vi "Set Data Name__ogtk.vi"(8 "error in (no error)":errorcluster, 9 "Data Name":string, 10 "Data":variant) -> (0 "error out":errorcluster, 2 "Renamed Data":variant)   [LabVIEW 2009]
doc: "Changes the Data Name of Variant Data.\n<b>Note:</b> Variant attributes will persist after this operation."
panel:
  # "Please visit http://www.OpenG.org to learn about the\nOpen Source LabVIEW software movement.\n\nNOTICE -- YOU MUST LEAVE THIS NOTICE IN PLACE.  PER THE TERMS OF THE LICENSE BELOW, YOU MAY SUBLICENSE THIS SOFTWARE \nIN ANY WAY THAT DOES NOT CONFLICT WITH THIS LICENSE.\n\n### BSD License (http://www.opensource.org/licenses/bsd-license.php) Begin ###\n \nCopyright (c) 2002, Jean-Pierre Drolet <drolet_jp@hotmail.com>\nCopyright (c) 2002-2006, Jim Kring <jim@jimkring.com>\nCopyright (c) 2011, Jonathon Green <jg@jgcode.net>\n\nAll rights reserved.\n\nRedistribution and use in source and binary forms, with or without modification, are permitted provided that the following conditions are met:\n\n    * Redistributions of source code must retain the above copyright notice, this list of conditions and the following disclaimer.\n    * Redistributions in binary form must reproduce the above copyright notice, this list of conditions and the following disclaimer in the \n       documentation and/or other materials provided with the distribution.\n    * Neither the name of SciWare, James Kring, Inc., nor the names of its contributors may be used to endorse or promote products derived \n       from this software without specific prior written permission.\n\nTHIS SOFTWARE IS PROVIDED BY THE COPYRIGHT HOLDERS AND CONTRIBUTORS \"AS IS\" AND ANY EXPRESS OR IMPLIED WARRANTIES, \nINCLUDING, BUT NOT LIMITED TO, THE IMPLIED WARRANTIES OF MERCHANTABILITY AND FITNESS FOR A PARTICULAR PURPOSE ARE \nDISCLAIMED. IN NO EVENT SHALL THE COPYRIGHT OWNER OR CONTRIBUTORS BE LIABLE FOR ANY DIRECT, INDIRECT, INCIDENTAL,\n SPECIAL, EXEMPLARY, OR CONSEQUENTIAL DAMAGES (INCLUDING, BUT NOT LIMITED TO, PROCUREMENT OF SUBSTITUTE GOODS OR \nSERVICES; LOSS OF USE, DATA, OR PROFITS; OR BUSINESS INTERRUPTION) HOWEVER CAUSED AND ON ANY THEORY OF LIABILITY, \nWHETHER IN CONTRACT, STRICT LIABILITY, OR TORT (INCLUDING NEGLIGENCE OR OTHERWISE) ARISING IN ANY WAY OUT OF THE USE \nOF THIS SOFTWARE, EVEN IF ADVISED OF THE POSSIBILITY OF SUCH DAMAGE.\n\n### BSD License End ###"
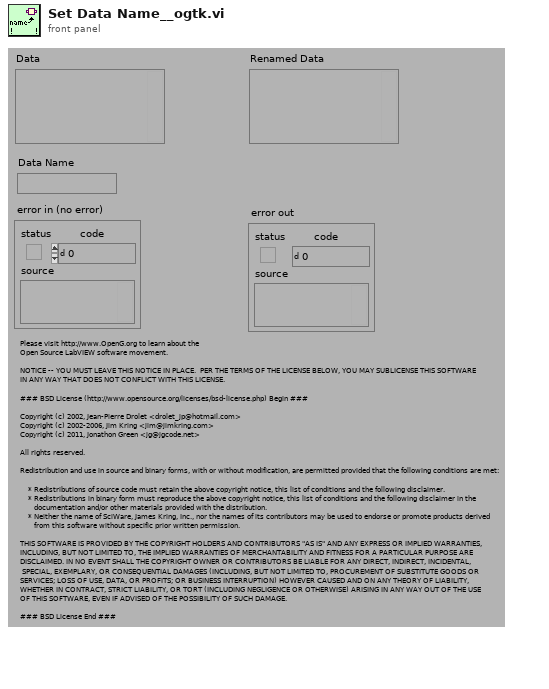
[diagram p1: front panel]
types:
  T1 = typedef "Type Descriptor Header__ogtk.ctl" = cluster{"length":u16, "private":u8, "type":T2, "# elements":u16}
  T2 = typedef "Type Descriptor Enumeration__ogtk.ctl" = enum8{"<Null>", "I8", "I16", "I32", "I64", "U8", "U16", "U32", "U64", "SGL", "DBL", "EXT", "CSG", "CDB", "CXT", "0x0F", "0x10", "0x11", "0x12", "0x13", "0x14", "Enum U8", "Enum U16", "Enum U32", "Enum U64", "SGL PQ", "DBL PQ", "EXT PQ", "CSG PQ", "CDB PQ", "CXT PQ", "0x1F", "0x20", "Boolean", "0x22", "0x23", "0x24", "0x25", "0x26", "0x27", "0x28", "0x29", "0x2A", "0x2B", "0x2C", "0x2D", "0x2E", "0x2F", "String", "0x31", "Path", "Pict", "0x34", "0x35", "0x36", "DAQ", "0x38", "0x39", "0x3A", "0x3B", "0x3C", "0x3D", "0x3E", "0x3F", "Array", "0x41", "0x42", "0x43", "0x44", "0x45", "0x46", "0x47", "0x48", "0x49", "0x4A", "0x4B", "0x4C", "0x4D", "0x4E", "0x4F", "Cluster", "0x51", "0x52", "Variant", "Waveform", "0x55", "0x56", "0x57", "0x58", "0x59", "0x5A", "0x5B", "0x5C", "0x5D", "0x5E", "0x5F", "0x60", "0x61", "0x62", "0x63", "0x64", "0x65", "0x66", "0x67", "0x68", "0x69", "0x6A", "0x6B", "0x6C", "0x6D", "0x6E", "0x6F", "Refnum"}
  T3 = typedef "Type Descriptor__ogtk.ctl" = i16[]
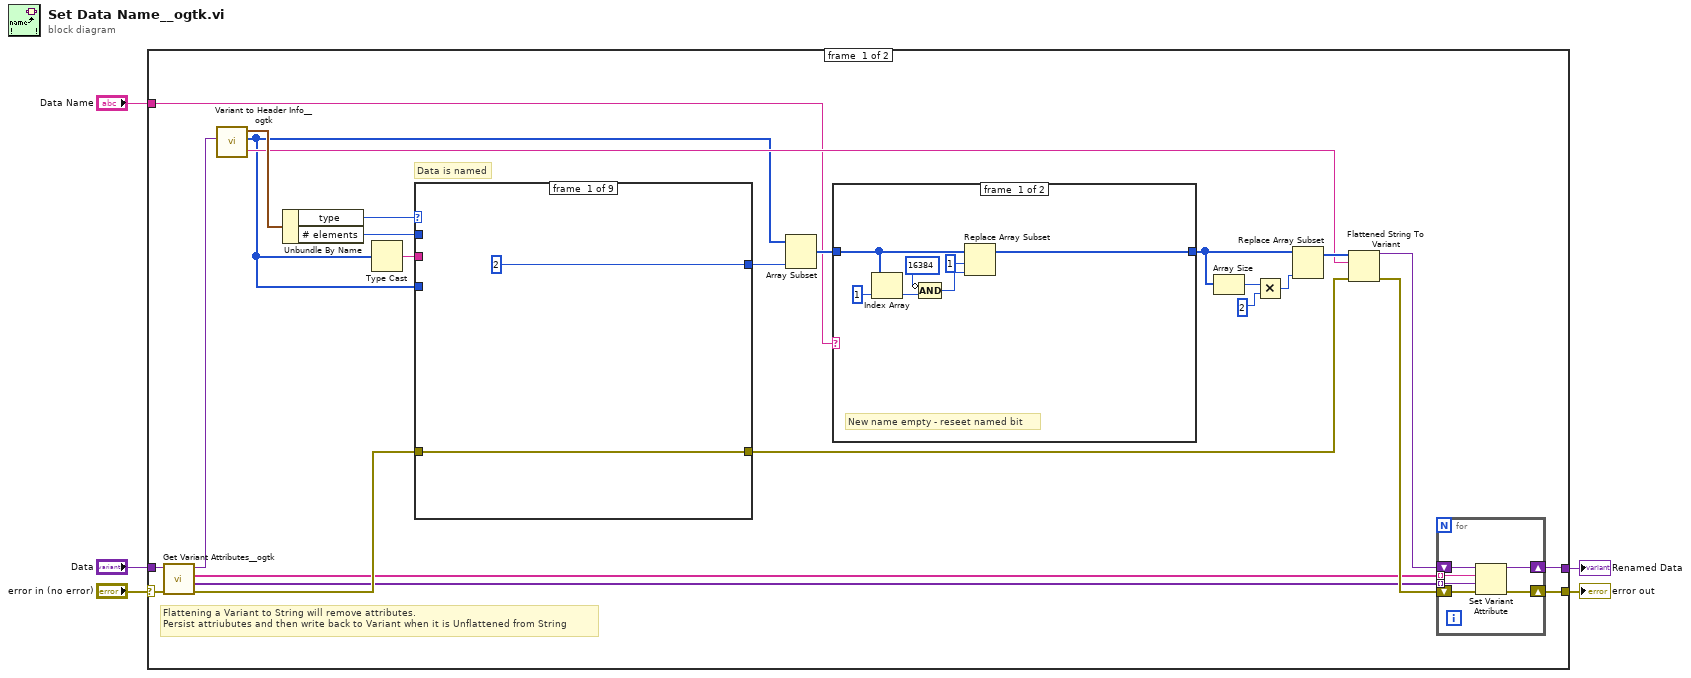
[diagram p0: block diagram]
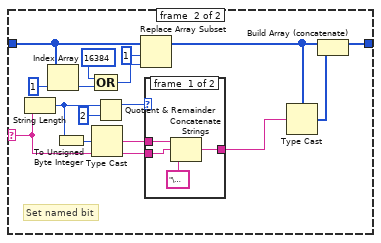
[diagram p2: hidden frame]
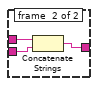
[diagram p3: hidden frame]
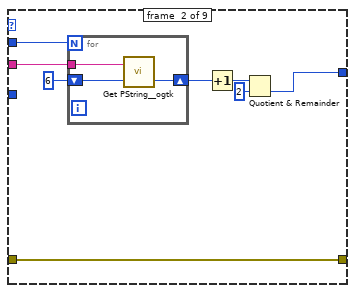
[diagram p4: hidden frame]
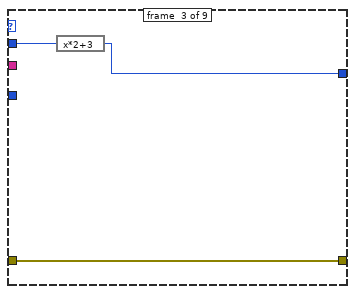
[diagram p5: hidden frame]
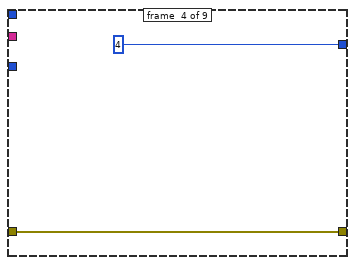
[diagram p6: hidden frame]
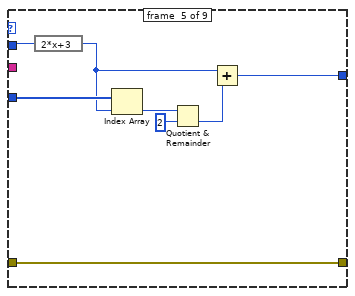
[diagram p7: hidden frame]
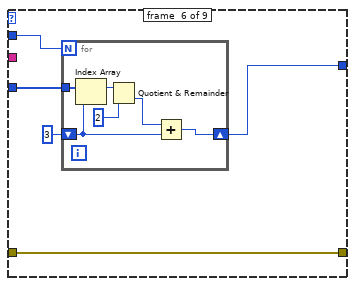
[diagram p8: hidden frame]
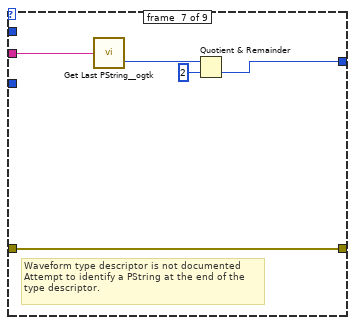
[diagram p9: hidden frame]
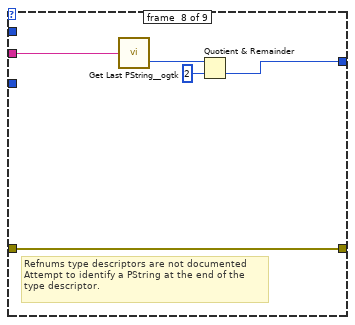
[diagram p10: hidden frame]
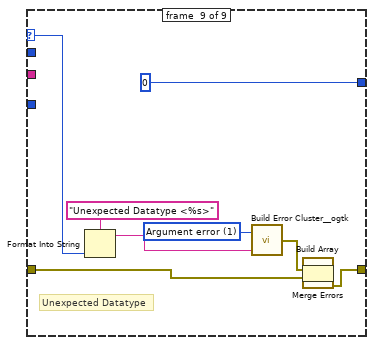
[diagram p11: hidden frame]
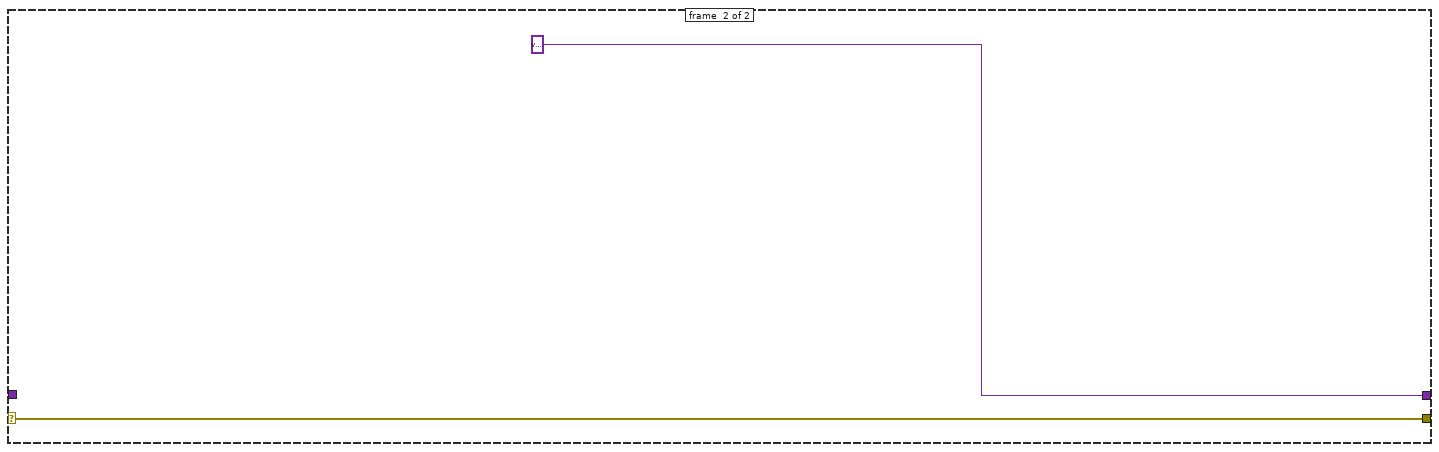
[diagram p12: hidden frame]
diagram:
  n1 = case shown="No Error" "error in (no error)" {
    selector: "error in (no error)" -> [w13 w124]
    tunnel: [w10 w124] -> w5
    tunnel: [w6 variant ("Renamed Data")] -> w3
    tunnel: "Data Name" -> [w16 _]
    tunnel: "Data" -> [w15 _]
    frame #0 {
      # "Flattening a Variant to String will remove attributes.\nPersist attriubutes and then write back to Variant when it is Unflattened from String"
      # "Data is named"
      n2 = call "Get Variant Attributes__ogtk.vi"("error in"=w13, "Variant"=w15) -> ("error out"=w12:errorcluster, "value(s)"=w9:variant[], "names"=w8:string[], "duplicate Variant"=w14:variant)  [unwired: 2 in]
      n3 = call "Variant to Header Info__ogtk.vi"("Variant"=w14) -> ("Type Descriptor Header"=w30:T1, "Type Descriptor"=w17:T3, "data string"=w19:string)  [unwired: 3 in]
      n4 = Unbundle By Name(w30) -> ("type"=w29:T2, "# elements"=w27:u16)
      n5 = Type Cast(x=w17) -> (*(type *) &x=w28:string)  [unwired: 1 in]
      n6 = case shown="\"Enum U8\"..\"Enum U64\"" w29 {
        selector: w29 -> [_ _ _ _ _ _ _ _ w120]
        tunnel: [w67 w70 w80 w83 w85 w93 w104 w109 w115] -> w18
        tunnel: w28 -> [_ w69 _ _ _ _ w108 w113 _]
        tunnel: w27 -> [_ w74 w82 _ w92 w97 _ _ _]
        tunnel: w17 -> [_ _ _ _ w91 w96 _ _ _]
        tunnel: [2 ("offset (0)") w71 w81 4 ("offset (0)") w86 w94 w105 w110 0 ("PString Offset")] -> w26
        tunnel: w12 -> [w67 w70 w80 w83 w85 w93 w104 w109 w117]
        frame #0 {
        }
        frame #1 {
          n7 = for {
            N: w74 -> [_]
            tunnel: w69 -> [w77]
            shift-right: [w78] -> w75
            shift-left: 6 -> [w79]
            n8 = call "Get PString__ogtk.vi"("offset (0)"=w79, "String"=w77) -> ("offset past PString"=w78:i32)  [unwired: 1 out]
          }
          n9 = Increment(x=w75) -> (x+1=w72:i32)
          n10 = Quotient & Remainder(x=w72, y=2) -> (floor(x/y)=w71:i32)  [unwired: 1 out]
        }
        frame #2 {
          n11 = expression code="x*2+3"(w82) -> (w81:u16)
        }
        frame #3 {
        }
        frame #4 {
          n12 = expression code="2*x+3"(w92) -> (w87:u16)
          n13 = Index Array(array=w91, index=w87) -> (element=w89:i16)
          n14 = Quotient & Remainder(x=w89, y=u16 2) -> (floor(x/y)=w88:u16)  [unwired: 1 out]
          n15 = Add(x=w87, y=w88) -> (x+y=w86:u16)
        }
        frame #5 {
          n16 = for {
            N: w97 -> [_]
            shift-right: [w102] -> w94
            shift-left: i16 3 -> [w101]
            tunnel: w96 -> [w103]
            n17 = Index Array(array=w103, index=w101) -> (element=w99:i16)
            n18 = Quotient & Remainder(x=w99, y=i16 2) -> (floor(x/y)=w100:i16)  [unwired: 1 out]
            n19 = Add(x=w100, y=w101) -> (x+y=w102:i16)
          }
        }
        frame #6 {
          # "Waveform type descriptor is not documented\nAttempt to identify a PString at the end of the\ntype descriptor."
          n20 = call "Get Last PString__ogtk.vi"("String"=w108) -> ("PString Offset"=w106:i32)  [unwired: 1 out]
          n21 = Quotient & Remainder(x=w106, y=2) -> (floor(x/y)=w105:i32)  [unwired: 1 out]
        }
        frame #7 {
          # "Refnums type descriptors are not documented\nAttempt to identify a PString at the end of the\ntype descriptor."
          n22 = call "Get Last PString__ogtk.vi"("String"=w113) -> ("PString Offset"=w111:i32)  [unwired: 1 out]
          n23 = Quotient & Remainder(x=w111, y=2) -> (floor(x/y)=w110:i32)  [unwired: 1 out]
        }
        frame #8 {
          w122 = 1 items=["No error", "Argument error", "Memory is full", "Out of zone", "End of file", "File already open", "Generic file I/O error", "File not found", "File permission error", "Disk is full", "Duplicate path", "Too many files open", "System feature not enabled", "Resource file not found", "Cannot add resource", "Resource not found", "Image not found", "Image memory error", "Pen does not exist", "Config type invalid", "Config token not found", "Config parse error", "Config memory error", "Bad external code format", "Bad external code offset", "External code not present", "Null window", "Destroy window error", "Null menu", "Print aborted", "Bad print record", "Print driver error", "Windows error during printing", "Memory error during printing", "Print dialog error", "Generic print error", "Invalid device refnum", "Device not found", "Device parameter error", "Device unit error", "Cannot open device", "Device call aborted", "Generic error", "Cancelled by user", "Object ID too low", "Object ID too high", "Object not in heap", "Unknown heap", "Unknown object (invalid DefProc)", "Unknown object (DefProc not in table)", "Message out of range", "Invalid (null) method", "Unknown message", "Manager call not supported", "Bad address", "Network operation in progress", "Network operation timed out", "Connection is busy", "Network attribute not supported", "Network error", "Address in use", "System out of memory", "Connection aborted", "Connection refused", "Not connected", "Already connected", "Connection closed", "Initialization error (interapplication manager)", "Bad occurrence", "Wait on unbound occurrence handler", "Occurrence queue overflow", "Datalog type conflict", "Unused", "Unrecognized type (interapplication manager)", "Memory corrupt", "Failed to make temporary DLL", "Old CIN version", "Drag socket not found", "Failed to load drop-object", "Failed to register OLE object", "Failed to release OLE object", "Format specifier type mismatch", "Unknown format specifier", "Too few format specifiers", "Too many format specifiers", "Scan failed", "Newer CIN version", "Error converting to variant", "Runtime menu error", "Password tampered", "Variant attribute not found", "Incompatible variant data type", "Event data is not available", "Event Store is not present", "Occurrence is not found", "Event Queue is not created", "Event info is not available", "Refnum passed is NULL", "Error retrieving Class GUID", "Error retrieving CoClass GUID", "Error retrieving TypeLib GUID.", "Bad built application magic bytes.", "Specific driver is different from the specific driver associated with the Logical Name.", "There is no session opened to the class driver.", "Max Error", "MAX - Error with config objects", "MAX - Error loading configuration", "MAX - Group not supported"]
          # "Unexpected Datatype"
          n24 = Format Into String(format string="Unexpected Datatype <%s>" ("Format String"), w120) -> (resulting string=w119:string)  [unwired: 2 in, 1 out]
          n25 = call "Build Error Cluster__ogtk.vi"("String to Prepend to source (\"\")"=w119, "code"=w122) -> ("error out"=w116:errorcluster)
          n26 = Build Array(w116, w117) -> (w114:errorcluster[])
          n27 = call <vilib>:"Merge Errors.vi"("error array in"=w114) -> ("error out"=w115:errorcluster)  [unwired: 6 in]
        }
      }
      n28 = Array Subset(array=w17, length=w26) -> (w25:T3)  [unwired: 1 in]
      n29 = case shown="\"\"" w16 {
        selector: w16 -> [_ w51]
        tunnel: w25 -> [w43 w59]
        tunnel: [w38 w48] -> w21
        frame #0 {
          # "New name empty - reseet named bit"
          n30 = Index Array(array=w43, index=1 ("Index")) -> (element=w41:i16)
          n31 = Compound Arithmetic op=AND(invert i16 16384 ("Input"), w41) -> (w40:i16)
          n32 = Replace Array Subset(array=w43, new element=w40, index=1 ("Index")) -> (w38:T3)
        }
        frame #1 {
          # "Set named bit"
          n33 = String Length(string=w51) -> (length=w47:i32)
          n34 = Index Array(array=w59, index=1 ("Index")) -> (element=w55:i16)
          n35 = To Unsigned Byte Integer(number=w47) -> (unsigned 8bit integer=w46:u8)
          n36 = Type Cast(x=w46) -> (*(type *) &x=w45:string)  [unwired: 1 in]
          n37 = Compound Arithmetic op=OR(i16 16384 ("Input"), w55) -> (w57:i16)
          n38 = Quotient & Remainder(x=w47, y=2) -> (x-y*floor(x/y)=w53:i32)  [unwired: 1 out]
          n39 = Replace Array Subset(array=w59, new element=w57, index=1 ("Index")) -> (w49:T3)
          n40 = case shown="1" w53 {
            tunnel: [w63 w64] -> w52
            tunnel: w51 -> [w62 w65]
            tunnel: w45 -> [w60 w66]
            frame #0 {
              n41 = Concatenate Strings(w60, w62, "\u0000" ("Substring")) -> (w63:string)
            }
            frame #1 {
              n42 = Concatenate Strings(w66, w65) -> (w64:string)
            }
          }
          n43 = Type Cast(type=w49, x=w52) -> (*(type *) &x=w50:T3)
          n44 = Build Array (concatenate)(w49, w50) -> (w48:T3)
        }
      }
      n45 = Array Size(array=w21) -> (size(s)=w24:i32)
      n46 = Multiply(x=w24, y=2) -> (x*y=w22:i32)
      n47 = Replace Array Subset(array=w21, new element=w22) -> (w20:T3)  [unwired: 1 in]
      n48 = Flattened String To Variant(4:w18, 6:w19, 7:w20) -> (0:w11:errorcluster, 3:w7:variant)
      n49 = for {
        shift-right: [w35] -> w10
        shift-left: w11 -> [w36]
        tunnel: w9 -> [w34] mode=indexing
        tunnel: w8 -> [w33] mode=indexing
        shift-right: [w31] -> w6
        shift-left: w7 -> [w32]
        n50 = Set Variant Attribute(Variant=w32, name=w33, value=w34, error in=w36) -> (Variant out=w31:variant, error out=w35:errorcluster)  [unwired: 1 out]
      }
    }
    frame #1 {
    }
  }
  "error out" <- w5
  "Renamed Data" <- w3
